vi "READ ALL TCS v2.vi"() -> ()   [LabVIEW 2016]
uses:
  <vilib>/Platform/TimedLoop/XDataNode/timing_clust.ctl
  <vilib>/Platform/TimedLoop/XDataNode/nitl_modes.ctl
  <vilib>/Platform/TimedLoop/XDataNode/wakeup.ctl
  <vilib>/DAQmx/read.llb/DAQmx Read (Analog 1D DBL NChan 1Samp).vi
  <vilib>/DAQmx/miscellaneous.llb/DAQmx Fill In Error Info.vi
  <vilib>/platform/TimedLoop/XDataNode/XDataNode.xnode
  <vilib>/Platform/TimedLoop/XDataNode/XDNodeRunTimeDep.lvlib
panel:
  out "Debugging":dbl
  in  "Write Data":bool
  out "TC Active?":T1
  in  "stop":bool
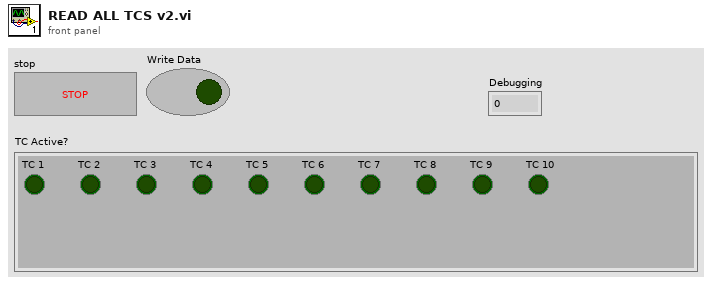
[diagram p1: front panel]
types:
  T1 = cluster{"TC 1":bool, "TC 2":bool, "TC 3":bool, "TC 4":bool, "TC 5":bool, "TC 6":bool, "TC 7":bool, "TC 8":bool, "TC 9":bool, "TC 10":bool}
  T2 = typedef "XDNodeRunTimeDep.lvlib/timing_clust.ctl" = cluster{"Expected End [f-1]":u64, "Actual End [f-1]":u64, "Finished Late? [f-1]":bool, "Expected End [i-1]":u64, "Actual End [i-1]":u64, "Finished Late? [i-1]":bool, "Expected Start [i]":u64, "Actual Start [i]":u64, "Expected Start [f]":u64, "Actual Start [f]":u64, "Source Name":string, "Structure Name":string, "Period":i64, "Deadline":i64, "Offset":i64, "Start":i64, "Priority":i32, "Timeout":i32, "Mode":T3, "Wakeup Reason":T4, "Error":errorcluster, "Source Type":string, "Secondary Source Type":string, "Global End Time":u64, "Global Start Time":u64, "Frame Duration":u64, "Iteration Duration":u64, "Assigned CPU":i32, "I/O Scan Engine Mode":u32}
  T3 = typedef "XDNodeRunTimeDep.lvlib/nitl_modes.ctl" = enum32{"No Change", "Process missed periods, maintain original phase", "Discard missed periods, maintain original phase", "Process missed periods, ignore original phase", "Discard missed periods, ignore original phase"}
  T4 = typedef "XDNodeRunTimeDep.lvlib/wakeup.ctl" = enum32{"Normal", "Aborted", "Asynchronous wakeup", "Timing source error", "Timed loop error", "Timeout"}
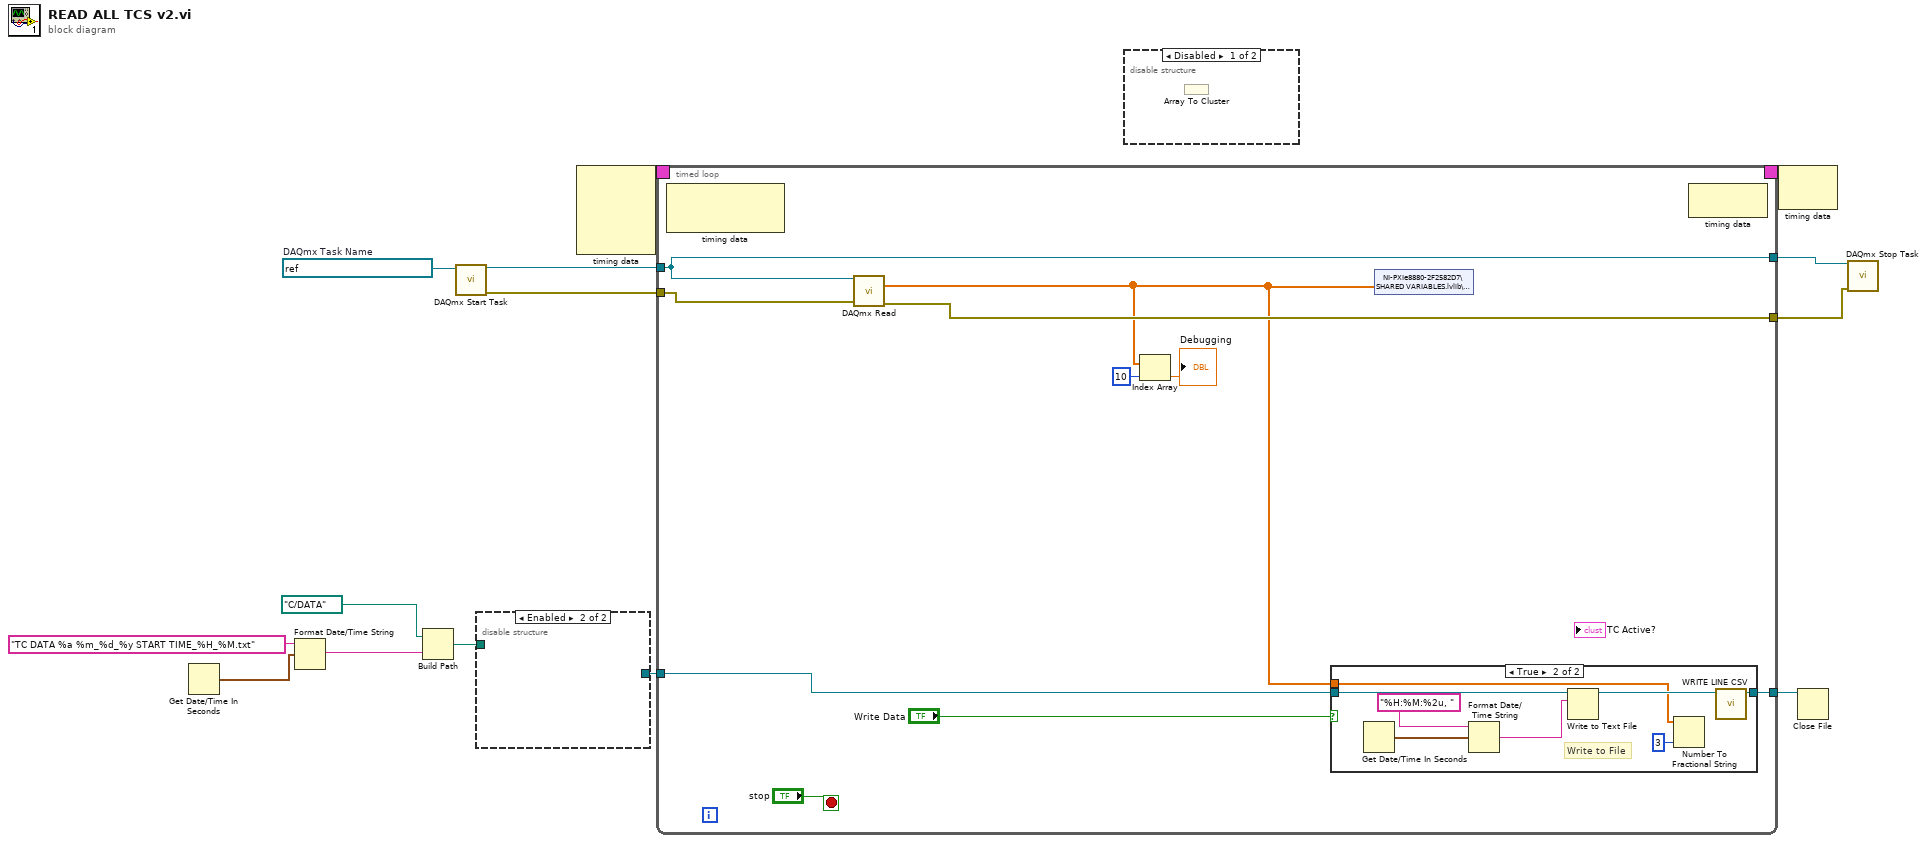
[diagram p0: block diagram]
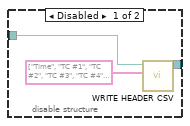
[diagram p3: hidden frame]
diagram:
  w14 = refnum<k21> "ALL THERMOCOUPLES"  # DAQmx Task Name
  n1 = Get Date/Time In Seconds() -> (seconds since 1Jan1904=w7:timestamp)
  n2 = Format Date/Time String(time format string (%c)="TC DATA %a %m_%d_%y START TIME_%H_%M.txt", seconds (now)=w7) -> (date/time string=w5:string)  [unwired: 1 in]
  n3 = Build Path(base path=path "C:/DATA", name or relative path=w5) -> (appended path=w4:path)
  n4 = call <vilib>:"DAQmx Start Task.vi"("task/channels in"=w14) -> ("task out"=w13:refnum<k21>, "error out"=w11:errorcluster)  [unwired: 13 in]
  n5 = disable-structure shown="Enabled" {
    disable-tunnel: [w16 _] -> w10
    disable-tunnel: w4 -> [w15 _]
    frame Disabled {
      n6 = call "WRITE HEADER CSV.vi"("Array"=string[] ["Time", "TC #1", "TC #2", "TC #3", "TC #4", "TC #5", "TC #6", "TC #7", "TC #8", "TC #9", "TC #10", "TC #11", "TC #12", "TC #13", "TC #14", "TC #15", "TC #16"], "file path"=w15) -> ("Byte Stream File out"=w16:refnum<file>)  [unwired: 9 in]
    }
    frame Enabled {
    }
  }
  n7 = node-c288() -> (w3:T2)  [unwired: 4 in]
  n8 = timed-loop {
    tunnel: w13 -> [w23]
    tunnel: [w23] -> w12
    tunnel: w11 -> [w22]
    tunnel: w10 -> [w25]
    tunnel: [w26] -> w9
    timing: w3 -> [_]
    timing-out: [_] -> w2
    tunnel: [w21] -> w1
    stop <- "stop" stop-if-true
    n9 = node-c288() -> ()  [unwired: 1 in, 2 out]
    n10 = call-poly <vilib>:"DAQmx Read.vi"("task/channels in"=w23, "error in"=w22) -> ("data"=w19:dbl[], "error out"=w21:errorcluster)  [unwired: 11 in, 1 out]
    n11 = Index Array(array=w19, index=10) -> (element=→"Debugging":dbl)
    n12 = case shown="True" "Write Data" {
      tunnel: [w30 w38] -> w26
      tunnel: w25 -> [w30 w34]
      tunnel: w19 -> [_ w31]
      frame False {
      }
      frame True {
        # "Write to File"
        n13 = Get Date/Time In Seconds() -> (seconds since 1Jan1904=w35:timestamp)
        n14 = Format Date/Time String(time format string (%c)="%H:%M:%2u, ", seconds (now)=w35) -> (date/time string=w33:string)  [unwired: 1 in]
        n15 = Write to Text File(file (use dialog)=w34, text=w33) -> (refnum out=w32:refnum<file>)  [unwired: 2 in, 2 out]
        n16 = Number To Fractional String(number=w31, precision (6)=i16 3) -> ()  [unwired: 2 in, 1 out]
        n17 = call "WRITE LINE CSV.vi"("FIle Ref"=w32) -> ("Byte Stream File out"=w38:refnum<file>)  [unwired: 10 in]
      }
    }
    n18 = shared-variable "NI-PXIe8880-2F2582D7\\SHARED VARIABLES.lvlib\\TC's Array"(w19) -> ()  [unwired: 1 in, 1 out]
    n19 = node-c288() -> ()  [unwired: 1 in, 1 out]
  }
  n20 = disable-structure shown="Disabled" {
    frame Disabled {
      n21 = Array To Cluster() -> ()  [unwired: 1 in, 1 out]
    }
    frame Enabled {
    }
  }
  n22 = node-c288(w2) -> ()  [unwired: 1 out]
  n23 = Close File(refnum=w9) -> ()  [unwired: 1 in, 2 out]
  n24 = call <vilib>:"DAQmx Stop Task.vi"("task/channels in"=w12, "error in"=w1) -> ()  [unwired: 12 in, 2 out]
